vi "Add Data without TS.vi"(8 "Error In":errorcluster, 10 "Values":dbl[](array[numeric]), 11 "BNT_XtGraph in":refnum<class "BNT_XtGraph.lvclass">) -> (0 "Error Out":errorcluster, 3 "BNT_XtGraph out":refnum<class "BNT_XtGraph.lvclass">)   [LabVIEW 2019, in "BNT_XtGraph.lvlib" / "BNT_XtGraph.lvclass"]
doc: "Add actual data with time <b>now</b> for all channels to history."
uses:
  BNT_XtGraph.lvclass
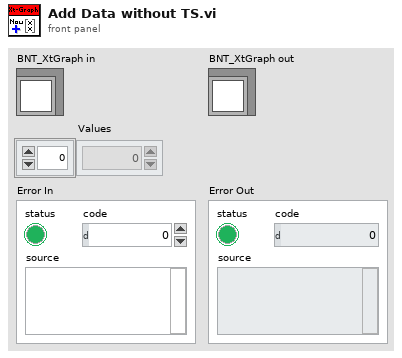
[diagram p1: front panel]
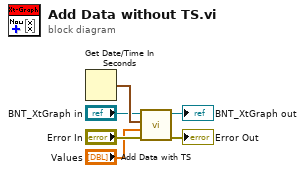
[diagram p0: block diagram]
diagram:
  n1 = Get Date/Time In Seconds() -> (seconds since 1Jan1904=w6:timestamp)
  n2 = call "Add Data with TS.vi"("Error In"="Error In", "Values"="Values", "Time Stamp"=w6, "BNT_XtGraph in"="BNT_XtGraph in") -> ("Error Out"=→"Error Out":errorcluster, "BNT_XtGraph out"=→"BNT_XtGraph out":refnum<class "BNT_XtGraph.lvclass">)  [unwired: 6 in]
